vi "format_to_uncertainty.vi"(8 "unit":string, 9 "Add SI prefix (true)":bool=TRUE, 10 "uncertainty":dbl format="%#_6p", 11 "value":dbl format="%#_6p") -> (0 "SI prefix and unit string":string, 1 "uncertainty format string":string, 2 "value format string":string, 3 "string out":string)   [LabVIEW 2013, in "varilib.lvlib"]
doc: "This VI combines value, uncertainty and unit into combined string formated to two significant digits. The VI also supports scaling by SI prefixes. Output format example: (1.0059 ± 0.0022) mV. SI prefix scaling can be disabled which may be usefull for unitless quantities."
uses:
  varilib.lvlib
  <vilib>/regexp/Match Regular Expression.xnode
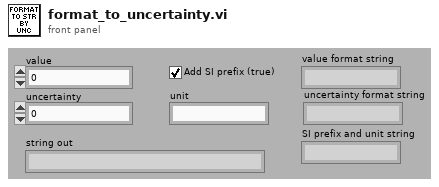
[diagram p1: front panel]
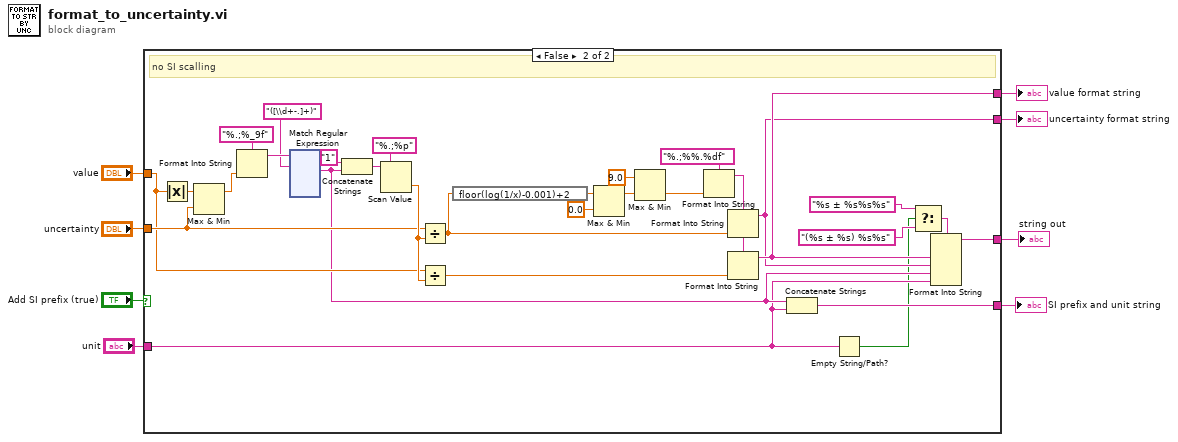
[diagram p0: block diagram]
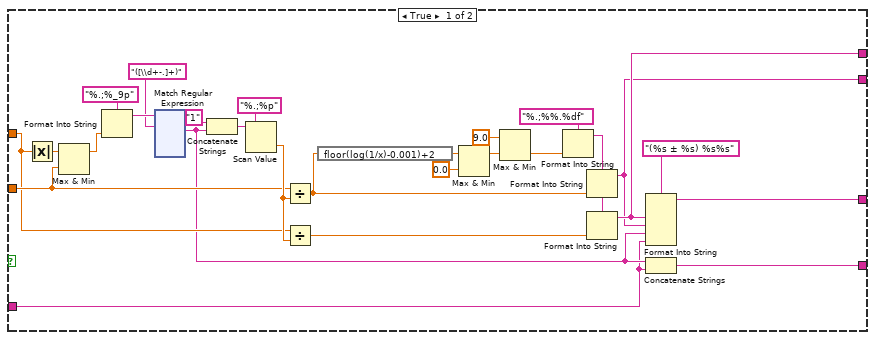
[diagram p2: hidden frame]
diagram:
  n1 = case shown="False" "Add SI prefix (true)" {
    tunnel: "value" -> [w20 w167]
    tunnel: "uncertainty" -> [w21 w168]
    tunnel: [w22 w169] -> w6
    tunnel: "unit" -> [w9 w153]
    tunnel: [w13 w160] -> w3
    tunnel: [w12 w159] -> w2
    tunnel: [w11 w157] -> w1
    frame True {
      n2 = Absolute Value(x=w20) -> (abs(x)=w17:dbl)
      n3 = Max & Min(x=w17, y=w21) -> (max(x,y)=w19:dbl)  [unwired: 1 out]
      n4 = Format Into String(format string="%.;%_9p", w19) -> (resulting string=w35:string)  [unwired: 2 in, 1 out]
      n5 = xnode "Match Regular Expression"("input string"=w35, "regular expression"="([\\d+-.]+)") -> ("after match"=w10:string)  [unwired: 4 in, 5 out]
      n6 = Concatenate Strings("1" ("string"), w10) -> (w32:string)
      n7 = Scan Value(string=w32, format string="%.;%p") -> (value=w28:dbl)  [unwired: 1 in, 1 out]
      n8 = Divide(x=w21, y=w28) -> (x/y=w26:dbl)
      n9 = Divide(x=w20, y=w28) -> (x/y=w27:dbl)
      n10 = expression code="floor(log(1/x)-0.001)+2"(w26) -> (w30:dbl)
      n11 = Max & Min(x=w30, y=0.0) -> (max(x,y)=w16:dbl)  [unwired: 1 out]
      n12 = Max & Min(x=9.0, y=w16) -> (min(x,y)=w15:dbl)  [unwired: 1 out]
      n13 = Format Into String(format string="%.;%%.%df", w15) -> (resulting string=w25:string)  [unwired: 2 in, 1 out]
      n14 = Format Into String(format string=w25, w26) -> (resulting string=w12:string)  [unwired: 2 in, 1 out]
      n15 = Format Into String(format string=w25, w27) -> (resulting string=w13:string)  [unwired: 2 in, 1 out]
      n16 = Format Into String(format string="(%s ± %s) %s%s", w13, w12, w10, w9) -> (resulting string=w22:string)  [unwired: 2 in, 1 out]
      n17 = Concatenate Strings(w10, w9) -> (w11:string)
    }
    frame False {
      # "no SI scalling"
      n18 = Absolute Value(x=w167) -> (abs(x)=w164:dbl)
      n19 = Max & Min(x=w164, y=w168) -> (max(x,y)=w166:dbl)  [unwired: 1 out]
      n20 = Format Into String(format string="%.;%_9f", w166) -> (resulting string=w181:string)  [unwired: 2 in, 1 out]
      n21 = xnode "Match Regular Expression"("input string"=w181, "regular expression"="([\\d+-.]+)") -> ("after match"=w158:string)  [unwired: 4 in, 5 out]
      n22 = Concatenate Strings("1" ("string"), w158) -> (w178:string)
      n23 = Scan Value(string=w178, format string="%.;%p") -> (value=w174:dbl)  [unwired: 1 in, 1 out]
      n24 = Divide(x=w168, y=w174) -> (x/y=w172:dbl)
      n25 = Divide(x=w167, y=w174) -> (x/y=w173:dbl)
      n26 = expression code="floor(log(1/x)-0.001)+2"(w172) -> (w176:dbl)
      n27 = Max & Min(x=w176, y=0.0) -> (max(x,y)=w163:dbl)  [unwired: 1 out]
      n28 = Max & Min(x=9.0, y=w163) -> (min(x,y)=w162:dbl)  [unwired: 1 out]
      n29 = Format Into String(format string="%.;%%.%df", w162) -> (resulting string=w171:string)  [unwired: 2 in, 1 out]
      n30 = Format Into String(format string=w171, w172) -> (resulting string=w159:string)  [unwired: 2 in, 1 out]
      n31 = Format Into String(format string=w171, w173) -> (resulting string=w160:string)  [unwired: 2 in, 1 out]
      n32 = Concatenate Strings(w158, w153) -> (w157:string)
      n33 = Empty String/Path?(string/path=w153) -> (empty?=w152:bool)
      n34 = Select(t="%s ± %s%s%s" ("format string"), s=w152, f="(%s ± %s) %s%s" ("format string")) -> (s? t:f=w156:string)
      n35 = Format Into String(format string=w156, w160, w159, w158, w153) -> (resulting string=w169:string)  [unwired: 2 in, 1 out]
    }
  }
  "string out" <- w6
  "value format string" <- w3
  "uncertainty format string" <- w2
  "SI prefix and unit string" <- w1
